vi "Detect Serial Break Event.vi"() -> ()   [LabVIEW 2023]
doc: "This example illustrates how to detect a break in the data line during serial communication. The VISA Enable Event function is used to enable an event for a serial break. The VISA Wait on Event function is used to wait for a break.\n\nThe serial port can set a serial break on the transmission lines. The serial port can detect that a serial break has occurred through the use of VISA Events. These events are notifications that allow a user to take action once the events have been detected. Note that all platforms allow the serial port to assert a break and receive notification of IO completion. However, the other serial events are valid only on Windows and platforms on which National Instruments supports ENET serial products. \n\nThis example shows how the user can detect that the break character has come across the transmission lines. The serial break event is specified by x3FFF2023. First, the event is enabled with VISA Enable Event, and any events already in the queue are discarded using VISA Discard Events. Then, VISA Wait on Event waits for the event type specified, in this case the x3FFF2023 or serial break event. VISA Wait on Event will wait for the specified timeout period. The expected VISA timeout error is -1073807339 (xBFFF0015). For the example, this timeout is ignored, so that the user has adequate time to see a break event detected. Also for this example, the number of breaks detected is displayed."
uses:
  support/Serial - Settings.ctl
  <vilib>/Instr/_visa.llb/Select Event Type.ctl
  <vilib>/Instr/_visa.llb/VISA Configure Serial Port (Instr).vi
panel:
  in  "Serial Settings":T1={"baud rate"=9600, "data bits"=8, "parity"=enum."None", "stop bits"=10, "flow control"=0} {"flow control" items=["None"=0, "XON/XOFF"=1, "RTS/CTS"=2, "DTR/DSR"=4]; "stop bits" items=["1.0"=10, "1.5"=15, "2.0"=20]; "data bits" min=5 max=8 step=1; "baud rate" items=["75"=75, "110"=110, "134"=134, "150"=150, "300"=300, "600"=600, "1200"=1200, "1800"=1800, "2400"=2400, "4800"=4800, "7200"=7200, "9600"=9600, "14400"=14400, "19200"=19200, "28800"=28800, "38400"=38400, "56000"=56000, "57600"=57600, "115200"=115200, "128000"=128000, "230400"=230400]}
  out "Number of Breaks":u32
  out "Timeout?":bool
  in  "Stop":bool
  out "Break Detected?":bool
  in  "VISA resource name":refnum<visa-resource-name>="COM1"
  # "Overview: Demonstrates the use of the VISA functions to detect a break in the line during serial communication.\nRequirements: NI-VISA Driver, multiple serial ports\nInstructions:\n1. Run the VI.\n2. Ensure Set Serial Break Event.vi is already running and follow the instructions on its front panel.\n3. Click Stop to stop the VI."
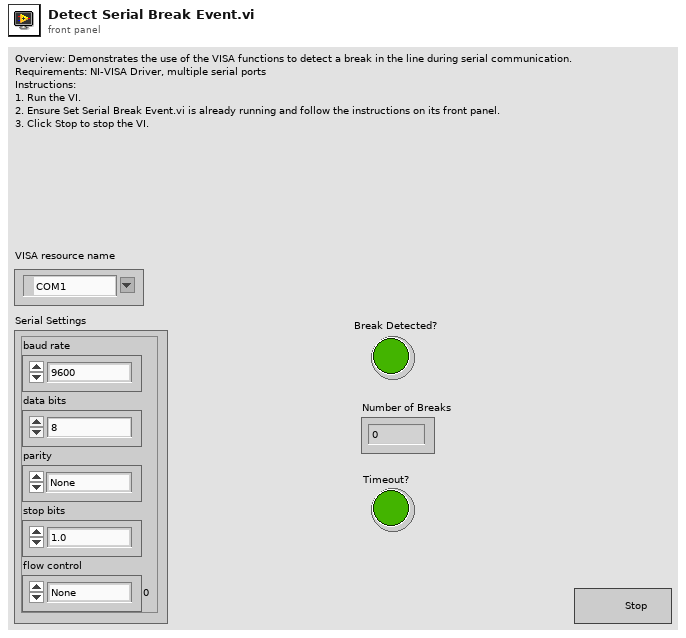
[diagram p1: front panel]
types:
  T1 = typedef "Serial - Settings.ctl" = cluster{"baud rate":u32, "data bits":u16, "parity":enum16{"None", "Odd", "Even", "Mark", "Space"}, "stop bits":u16, "flow control":u16}
  T2 = typedef "Select Event Type.ctl" = u32
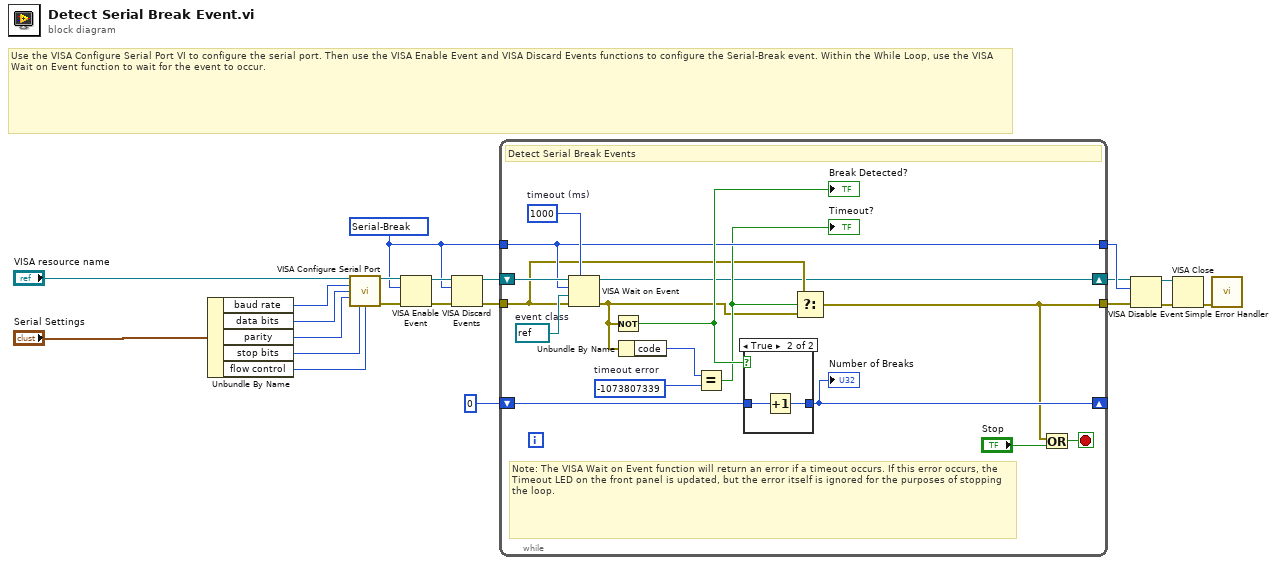
[diagram p0: block diagram]
diagram:
  w13 = T2 1073684515 items=["ServiceRequest"=1073684491, "Trigger"=3221168138, "Clear"=1073684493, "VXI-Signal"=1073684512, "VXI/VME-Interrupt"=3221168161, "VXI/VME-Sysfail"=1073684509, "VXI/VME-Sysreset"=1073684510, "GPIB-CIC"=1073684498, "GPIB-Talk"=1073684499, "GPIB-Listen"=1073684500, "PXI-Interrupt"=1073684514, "AllEnabled"=1073709055, "Serial-Break"=1073684515, "Serial-TermChar"=1073684516, "Serial-CTS"=1073684521, "Serial-DSR"=1073684522, "Serial-DCD"=1073684524, "Serial-RI"=1073684526, "Serial-Character"=1073684533] ("Event Type")
  # "Use the VISA Configure Serial Port VI to configure the serial port. Then use the VISA Enable Event and VISA Discard Events functions to configure the Serial-Break event. Within the While Loop, use the VISA Wait on Event function to wait for the event to occur."
  n1 = Unbundle By Name("Serial Settings") -> ("baud rate"=w6:u32, "data bits"=w5:u16, "parity"=w4:enum16{"None", "Odd", "Even", "Mark", "Space"}, "stop bits"=w3:u16, "flow control"=w2:u16)
  n2 = call-poly "VISA Configure Serial Port"("VISA resource name"="VISA resource name", "baud rate (9600)"=w6, "data bits (8)"=w5, "parity (0:none)"=w4, "stop bits (10: 1 bit)"=w3, "flow control (0:none)"=w2) -> ("VISA resource name out"=w19:refnum<visa-resource-name>, "error out"=w16:errorcluster)  [unwired: 3 in, 5 out]
  n3 = VISA Enable Event(8:w16, 10:w13, 11:w19) -> (0:w15:errorcluster, 3:w18:refnum<visa-resource-name>)  [unwired: 1 out]
  n4 = VISA Discard Events(8:w15, 10:w13, 11:w18) -> (0:w14:errorcluster, 3:w17:refnum<visa-resource-name>)  [unwired: 1 out]
  n5 = while {
    tunnel: w14 -> [w25]
    tunnel: [w23] -> w11
    shift-right: [w32] -> _
    shift-left: u32 0 ("timeout (0)") -> [w33]
    tunnel: w13 -> [w29]
    tunnel: [w29] -> w9
    shift-right: [w22] -> w1
    shift-left: w17 -> [w30]
    stop <- w24 stop-if-true
    w28 = refnum<visa-resource-name> refnum  # event class
    w35 = -1073807339  # timeout error
    w37 = u32 1000  # timeout (ms)
    # "Note: The VISA Wait on Event function will return an error if a timeout occurs. If this error occurs, the Timeout LED on the front panel is updated, but the error itself is ignored for the purposes of stopping the loop."
    # "Detect Serial Break Events"
    n6 = VISA Wait on Event(7:w37, 8:w25, 9:w28, 10:w29, 11:w30) -> (0:w26:errorcluster, 3:w22:refnum<visa-resource-name>)  [unwired: 2 out]
    n7 = Not(x=w26) -> (.not. x?=w34:bool)
    "Break Detected?" <- w34
    n8 = Unbundle By Name(w26) -> ("code"=w36:i32)
    n9 = Equal?(x=w36, y=w35) -> (x = y?=w27:bool)
    "Timeout?" <- w27
    n10 = case shown="True" w34 {
      tunnel: w33 -> [w38 w40]
      tunnel: [w38 w39] -> w32
      frame False {
      }
      frame True {
        n11 = Increment(x=w40) -> (x+1=w39:u32)
      }
    }
    "Number of Breaks" <- w32
    n12 = Select(t=w25, s=w27, f=w26) -> (s? t:f=w23:errorcluster)
    n13 = Or(x=w23, y="Stop") -> (x .or. y?=w24:bool)
  }
  n14 = VISA Disable Event(8:w11, 10:w9, 11:w1) -> (0:w10:errorcluster, 3:w12:refnum<visa-resource-name>)  [unwired: 1 out]
  n15 = VISA Close(VISA resource name=w12, error in (no error)=w10) -> (error out=w8:errorcluster)
  n16 = call <vilib>:"Simple Error Handler.vi"("error in (no error)"=w8) -> ()  [unwired: 1 in, 8 out]
